vi "traceFileIO_readFromFile_multiple_idx.vi"(0 "reference in":refnum<class "OSA.lvclass">, 1 "path":path, 3 "dataType":T1, 4 "trace idx start":u32, 5 "error in (no error)":errorcluster, 7 "dialog (empty path)":bool) -> (14 "reference out":refnum<class "OSA.lvclass">, 16 "traces nr":i32, 18 "cancelled":bool, 19 "error out":errorcluster)   [LabVIEW 2010, in "OSA.lvclass"]
doc: "Checks nr of traces in file and updates required nr of trace buffers. \n\nSupported fileformat: spf2.\n\nPlease note; traces saved from the application GUI will not load accurately!"
uses:
  OSA.lvclass
  typeDef/acq_dataType.ctl
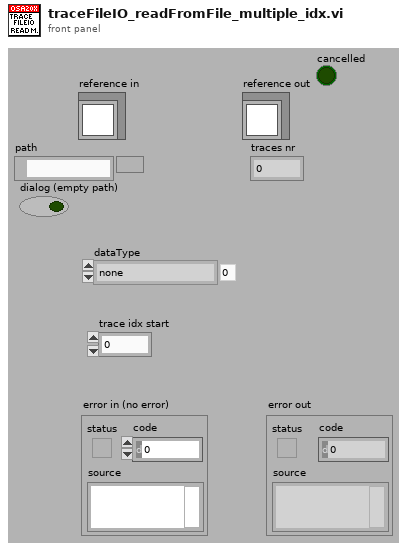
[diagram p1: front panel]
types:
  T1 = typedef "OSA.lvclass/acq_dataType.ctl" = enum16{"none", "interferogram", "spectrum"}
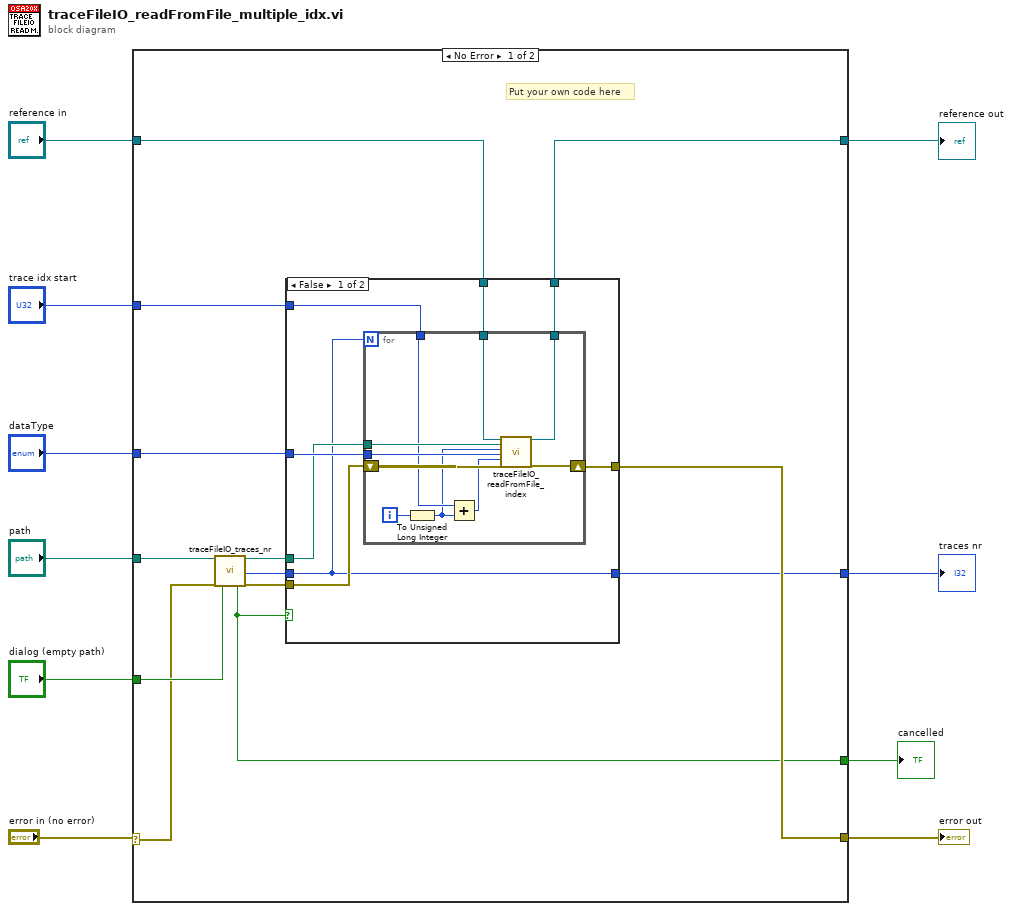
[diagram p0: block diagram]
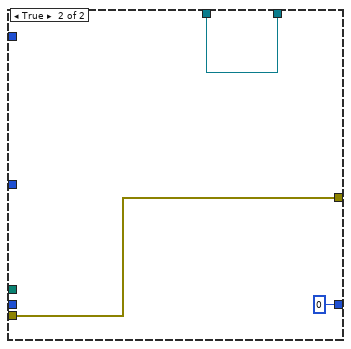
[diagram p2: hidden frame]
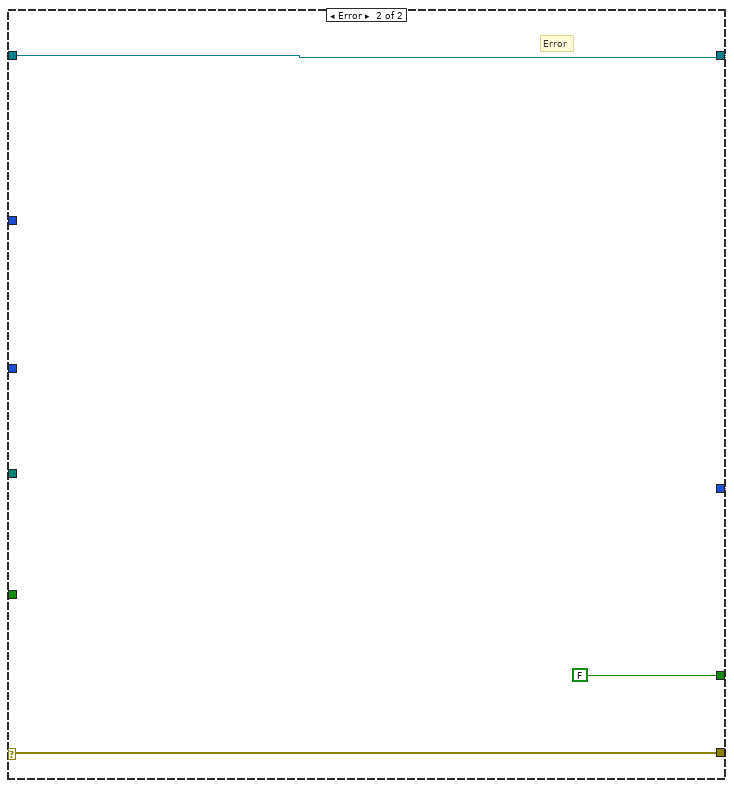
[diagram p3: hidden frame]
diagram:
  n1 = case shown="No Error" "error in (no error)" {
    selector: "error in (no error)" -> [w16 w48]
    tunnel: [w13 w48] -> w10
    tunnel: "reference in" -> [w17 w47]
    tunnel: [w19 w47] -> w5
    tunnel: "dataType" -> [w20 _]
    tunnel: "trace idx start" -> [w14 _]
    tunnel: "path" -> [w23 _]
    tunnel: "dialog (empty path)" -> [w22 _]
    tunnel: [w12 0 ("traces nr")] -> w2
    tunnel: [w11 FALSE ("cancelled")] -> w1
    frame No Error {
      # "Put your own code here"
      n2 = call "traceFileIO_traces_nr.vi"("path"=w23, "error in (no error)"=w16, "dialog (empty path)"=w22) -> ("cancelled"=w11:bool, "actual path"=w15:path, "traces nr"=w18:i32, "error out"=w21:errorcluster)  [unwired: 13 in]
      n3 = case shown="False" w11 {
        tunnel: w21 -> [w29 w42]
        tunnel: w20 -> [w28 _]
        tunnel: w14 -> [w26 _]
        tunnel: w17 -> [w31 w44]
        tunnel: [w30 w44] -> w19
        tunnel: w18 -> [w24 _]
        tunnel: w15 -> [w27 _]
        tunnel: [w25 w42] -> w13
        tunnel: [w24 0 ("traces nr")] -> w12
        frame False {
          n4 = for {
            N: w24 -> [_]
            tunnel: w31 -> [w41]
            tunnel: [w40] -> w30
            shift-right: [w38] -> w25
            shift-left: w29 -> [w39]
            tunnel: w28 -> [w37]
            tunnel: w27 -> [w36]
            tunnel: w26 -> [w35]
            i -> [w33]
            n5 = To Unsigned Long Integer(number=w33) -> (unsigned 32bit integer=w32:u32)
            n6 = Add(x=w35, y=w32) -> (x+y=w34:u32)
            n7 = call "traceFileIO_readFromFile_index.vi"("reference"=w41, "path"=w36, "file_trace idx"=w32, "dataType"=w37, "trace idx"=w34, "error in (no error)"=w39) -> ("duplicate reference"=w40:refnum<class "OSA.lvclass">, "error out"=w38:errorcluster)  [unwired: 11 in, 1 out]
          }
        }
        frame True {
        }
      }
    }
    frame Error {
      # "Error"
    }
  }
  "error out" <- w10
  "reference out" <- w5
  "traces nr" <- w2
  "cancelled" <- w1
